vi "04 LV - Run lifecycle.vi"   [LabVIEW 2020]
uses:
  d88b689d-885a-40c2-99c3-e80819a83aad.vi
  client/Client/Client.lvclass
  client/Asset/Asset.lvclass
  client/RunCreateStaging/RunCreateStaging.lvclass
  client/Run/Run.lvclass
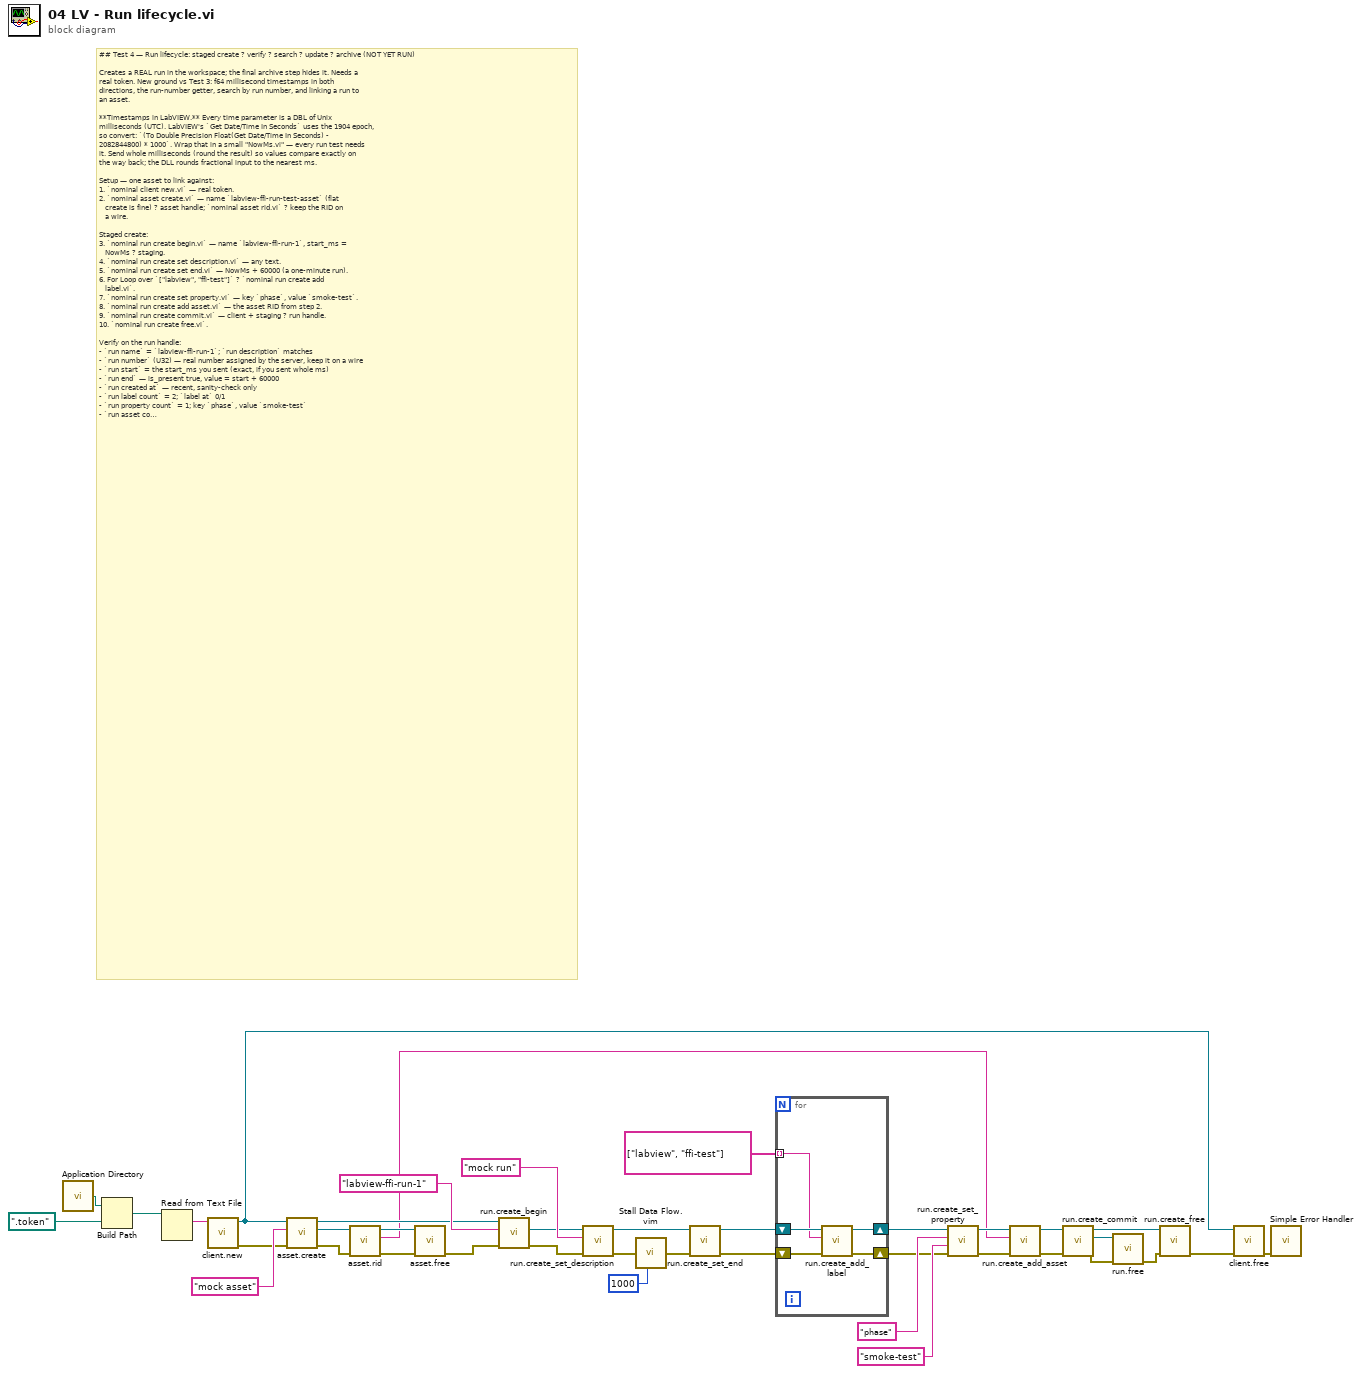
[diagram p0: block diagram]
diagram:
  # "## Test 4 — Run lifecycle: staged create ? verify ? search ? update ? archive (NOT YET RUN)\n\nCreates a REAL run in the workspace; the final archive step hides it. Needs a\nreal token. New ground vs Test 3: f64 millisecond timestamps in both\ndirections, the run-number getter, search by run number, and linking a run to\nan asset.\n\n**Timestamps in LabVIEW.** Every time parameter is a DBL of Unix\nmilliseconds (UTC). LabVIEW's `Get Date/Time In Seconds` uses the 1904 epoch,\nso convert: `(To Double Precision Float(Get Date/Time In Seconds) -\n2082844800) * 1000`. Wrap that in a small \"NowMs.vi\" — every run test needs\nit. Send whole milliseconds (round the result) so values compare exactly on\nthe way back; the DLL rounds fractional input to the nearest ms.\n\nSetup — one asset to link against:\n1. `nominal client new.vi` — real token.\n2. `nominal asset create.vi` — name `labview-ffi-run-test-asset` (flat\n   create is fine) ? asset handle; `nominal asset rid.vi` ? keep the RID on\n   a wire.\n\nStaged create:\n3. `nominal run create begin.vi` — name `labview-ffi-run-1`, start_ms =\n   NowMs ? staging.\n4. `nominal run create set description.vi` — any text.\n5. `nominal run create set end.vi` — NowMs + 60000 (a one-minute run).\n6. For Loop over `[\"labview\", \"ffi-test\"]` ? `nominal run create add\n   label.vi`.\n7. `nominal run create set property.vi` — key `phase`, value `smoke-test`.\n8. `nominal run create add asset.vi` — the asset RID from step 2.\n9. `nominal run create commit.vi` — client + staging ? run handle.\n10. `nominal run create free.vi`.\n\nVerify on the run handle:\n- `run name` = `labview-ffi-run-1`; `run description` matches\n- `run number` (U32) — real number assigned by the server, keep it on a wire\n- `run start` = the start_ms you sent (exact, if you sent whole ms)\n- `run end` — is_present true, value = start + 60000\n- `run created at` — recent, sanity-check only\n- `run label count` = 2; `label at` 0/1\n- `run property count` = 1; key `phase`, value `smoke-test`\n- `run asset count` = 1; `run asset rid at` 0 = the RID from step 2\n- `run rid` — keep on a wire; `run url` — optional browser check (URL uses\n  the run number, not the RID)\n\nSearch by run number (proves the non-string filters):\n11. `nominal run search.vi` — search_text/label/property empty, run_number =\n    the number from the verify step, has_start_after/has_end_before false ?\n    expect count = 1; `nominal handle list get` index 0 ? `run rid` matches;\n    free the run handle and the list.\n\nStaged update (replace semantics again):\n12. `nominal run update begin.vi` ? staging; `add label` `updated`;\n    `set end` NowMs + 120000.\n13. `nominal run update commit.vi` — client, run RID, staging ? new handle.\n14. `nominal run update free.vi`. On the NEW handle: `label count` = 1\n    (labels replaced), `end` = the new value, `start` unchanged.\n\nCleanup:\n15. `nominal run archive.vi` — client + run RID.\n16. `nominal asset archive.vi` — client + asset RID (from step 2).\n17. `nominal run free.vi` on both run handles, `nominal asset free.vi`,\n    `nominal client free.vi`."
  n1 = call <vilib>:"Application Directory.vi"() -> ("Application Directory"=w39:path)
  n2 = Build Path(base path=w39, name or relative path=path ".token") -> (appended path=w37:path)
  n3 = Read from Text File(file (use dialog)=w37) -> (text=w35:string)  [unwired: 3 in, 3 out]
  n4 = call "client.new.vi"("token"=w35) -> ("error out"=w27:errorcluster, "Client out"=w33:refnum<class "Client.lvclass">)  [unwired: 9 in]
  n5 = call "asset.create.vi"("error in"=w27, "name"="mock asset", "Client in"=w33) -> ("error out"=w30:errorcluster, "Asset"=w31:refnum<class "Asset.lvclass">, "Client out"=w24:refnum<class "Client.lvclass">)  [unwired: 6 in]
  n6 = call "asset.rid.vi"("error in"=w30, "asset in"=w31) -> ("error out"=w28:errorcluster, "RID"=w9:string, "asset out"=w29:refnum<class "Asset.lvclass">)  [unwired: 7 in]
  n7 = call "asset.free.vi"("error in"=w28, "asset in"=w29) -> ("error out"=w25:errorcluster)  [unwired: 9 in]
  n8 = call "run.create_begin.vi"("error in"=w25, "Name"="labview-ffi-run-1" ("name"), "Client in"=w24) -> ("error out"=w21:errorcluster, "RunCreateStaging"=w22:refnum<class "RunCreateStaging.lvclass">)  [unwired: 6 in, 1 out]
  n9 = call "run.create_set_description.vi"("error in"=w21, "description"="mock run" ("name"), "RunCreateStaging in"=w22) -> ("error out"=w19:errorcluster, "RunCreateStaging out"=w20:refnum<class "RunCreateStaging.lvclass">)  [unwired: 7 in]
  n10 = call "Stall Data Flow.vim"("value in"=w19, "milliseconds to wait"=u32 1000) -> ("value out"=w17:errorcluster)  [unwired: 1 out]
  n11 = call "run.create_set_end.vi"("error in"=w17, "RunCreateStaging in"=w20) -> ("error out"=w15:errorcluster, "RunCreateStaging out"=w18:refnum<class "RunCreateStaging.lvclass">)  [unwired: 8 in]
  n12 = for {
    tunnel: string[] ["labview", "ffi-test"] ("name") -> [w42] mode=indexing
    shift-right: [w40] -> w12
    shift-left: w15 -> [w41]
    shift-right: [w44] -> w11
    shift-left: w18 -> [w43]
    n13 = call "run.create_add_label.vi"("error in"=w41, "label"=w42, "RunCreateStaging in"=w43) -> ("error out"=w40:errorcluster, "RunCreateStaging out"=w44:refnum<class "RunCreateStaging.lvclass">)  [unwired: 7 in]
  }
  n14 = call "run.create_set_property.vi"("error in"=w12, "value"="smoke-test" ("name"), "key"="phase" ("name"), "RunCreateStaging in"=w11) -> ("error out"=w8:errorcluster, "RunCreateStaging out"=w10:refnum<class "RunCreateStaging.lvclass">)  [unwired: 6 in]
  n15 = call "run.create_add_asset.vi"("error in"=w8, "asset_rid"=w9, "RunCreateStaging in"=w10) -> ("error out"=w6:errorcluster, "RunCreateStaging out"=w7:refnum<class "RunCreateStaging.lvclass">)  [unwired: 7 in]
  n16 = call "run.create_commit.vi"("error in"=w6, "RunCreateStaging in"=w7) -> ("error out"=w2:errorcluster, "Run"=w3:refnum<class "Run.lvclass">, "RunCreateStaging out"=w5:refnum<class "RunCreateStaging.lvclass">)  [unwired: 7 in]
  n17 = call "run.free.vi"("error in"=w2, "Run in"=w3) -> ("error out"=w1:errorcluster)  [unwired: 9 in]
  n18 = call "run.create_free.vi"("error in"=w1, "RunCreateStaging"=w5) -> ("error out"=w4:errorcluster)  [unwired: 9 in]
  n19 = call "client.free.vi"("error in"=w4, "Client in"=w33) -> ("error out"=w34:errorcluster)  [unwired: 9 in]
  n20 = call <vilib>:"Simple Error Handler.vi"("error in (no error)"=w34) -> ()  [unwired: 4 in, 5 out]
